vi "clearError.vi"(8 "error in (no error)":errorcluster, 10 "model in":refnum<class "IModel.lvclass">, 11 "FaultState in":refnum<class "FaultState.lvclass">) -> (0 "error out":errorcluster, 2 "model out":refnum<class "IModel.lvclass">, 3 "FaultState out":refnum<class "FaultState.lvclass">)   [LabVIEW 2015, in "States.lvlib" / "FaultState.lvclass"]
uses:
  FaultState.lvclass
  IModel/IModel.lvclass
  Typedefs/StateValue.ctl
  ComponentTemplateCore/ComponentModel/ComponentModel/Typedefs/ComponentStateValues.ctl
  ComponentTemplateCore/ComponentModel/ComponentModel/InternalSignals/clearMessagingError.vi
  Typedefs/EXATypedefs.lvlib
  ComponentTemplateCore/ComponentModel/ComponentModel/InternalSignals/InternalSignalsGlobals.lvlib
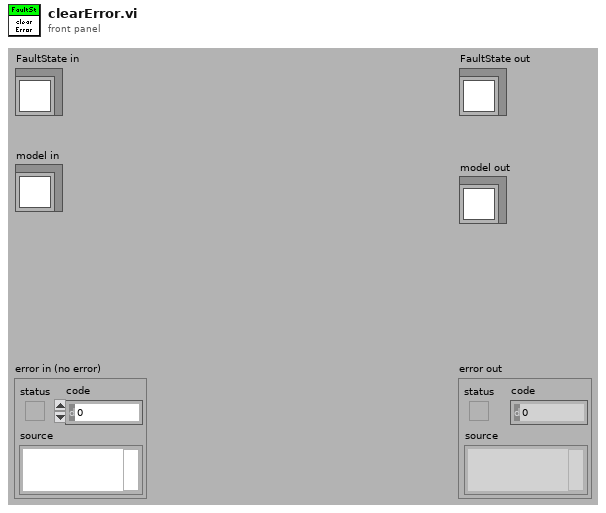
[diagram p1: front panel]
types:
  T1 = typedef "componentStateValues.ctl" = enum16{"Off", "Standby", "Enabled", "Disabled", "Fault"}
  T2 = typedef "EXATypedefs.lvlib/StateValue.ctl" = enum16{"DisabledState", "EnabledState", "FaultState", "OffState", "StandbyState"}
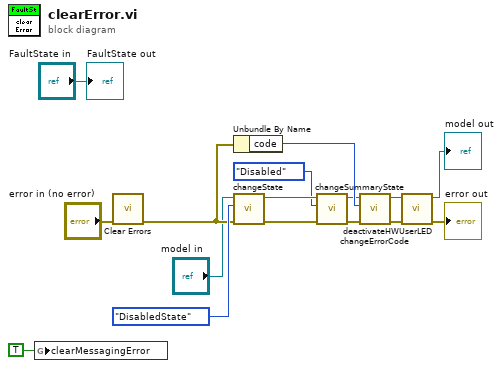
[diagram p0: block diagram]
diagram:
  n1 = global write "clearMessagingError.vi" "clearMessagingError"(TRUE ("clearMessagingError")) -> ()
  n2 = call <vilib>:"Clear Errors.vi"("error in (no error)"="error in (no error)") -> ("error out"=w13:errorcluster)  [unwired: 5 in, 1 out]
  n3 = Unbundle By Name(w13) -> ("code"=w14:i32)
  n4 = call-dynamic "changeState.vi"("error in (no error)"=w13, "newState"=StateValue."DisabledState" ("DetailedStateValue"), "IModel in"="model in") -> ("error out"=w9:errorcluster, "IModel out"=w12:refnum<class "IModel.lvclass">)  [unwired: 7 in]
  n5 = call-dynamic "changeSummaryState.vi"("error in (no error)"=w9, "newSummaryState"=componentStateValues."Disabled" ("componentStateValues"), "IModel in"=w12) -> ("error out"=w8:errorcluster, "IModel out"=w11:refnum<class "IModel.lvclass">)  [unwired: 7 in]
  n6 = call-dynamic "changeErrorCode.vi"("error in (no error)"=w8, "error.code"=w14, "IModel in"=w11) -> ("error out"=w3:errorcluster, "IModel out"=w5:refnum<class "IModel.lvclass">)  [unwired: 7 in]
  n7 = call-dynamic "deactivateHWUserLED.vi"("error in (no error)"=w3, "IModel in"=w5) -> ("error out"=→"error out":errorcluster, "IModel out"=→"model out":refnum<class "IModel.lvclass">)  [unwired: 8 in]
  "FaultState out" <- "FaultState in"
